vi "Update Inverter Data in MeasDataQ.vi"(6 "UpdateTS (T)":bool=TRUE, 8 "error in (no error)":errorcluster, 9 "TimeStamp":timestamp, 11 "Inverter Data":T1) -> (0 "error out":errorcluster, 3 "InverterWaveformsQ out":T2)   [LabVIEW 2019]
doc: "Developed by Kevin Thompson\nThompson Engineering, LLC\nkevin@thompsonengineering.net"
uses:
  TD MeasData--cluster.ctl
  TD MeasData QRef.ctl
  GBL DataQ Ref.vi
  DataTypes/InverterData--cluster.ctl
  DataTypes/InverterPhaseData--cluster.ctl
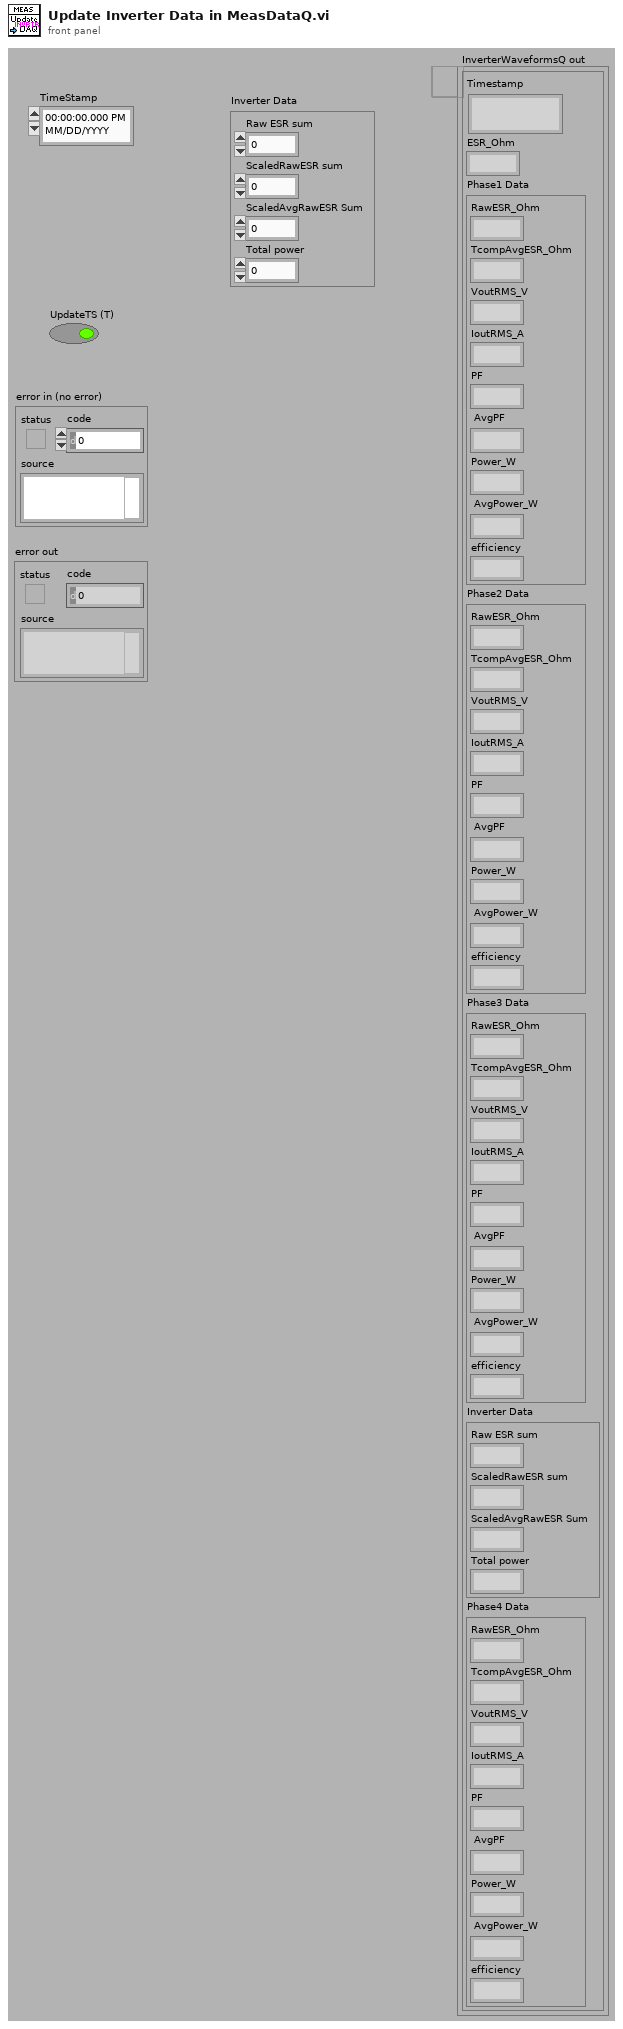
[diagram p1: front panel]
types:
  T1 = typedef "InverterData--cluster.ctl" = cluster{"Raw ESR sum":dbl, "ScaledRawESR sum":dbl, "ScaledAvgRawESR Sum":dbl, "Total power":dbl}
  T2 = typedef "TD MeasData QRef.ctl" = refnum<queue>
  T3 = typedef "TD MeasData--cluster.ctl" = cluster{"Timestamp":timestamp, "ESR_Ohm":dbl, "Phase1 Data":T4, "Phase2 Data":T4, "Phase3 Data":T4, "Inverter Data":T1, "Phase4 Data":T4}
  T4 = typedef "InverterPhaseData--cluster.ctl" = cluster{"RawESR_Ohm":dbl, "TcompAvgESR_Ohm":dbl, "VoutRMS_V":dbl, "IoutRMS_A":dbl, "PF":dbl, "AvgPF":dbl, "Power_W":dbl, "AvgPower_W":dbl, "efficiency":dbl}
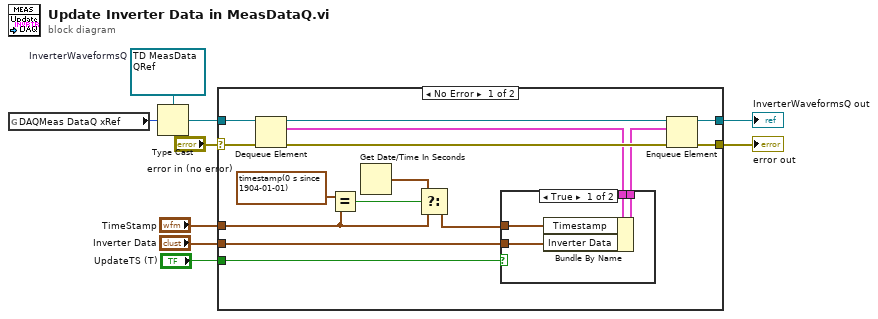
[diagram p0: block diagram]
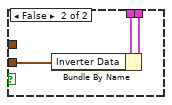
[diagram p2: hidden frame]
diagram:
  w6 = T2 refnum  # InverterWaveformsQ
  n1 = global read "GBL DataQ Ref.vi" "DAQMeas DataQ xRef"() -> (w3:u32)
  n2 = Type Cast(type=w6, x=w3) -> (*(type *) &x=w5:T2)
  n3 = case shown="No Error" "error in (no error)" {
    selector: "error in (no error)" -> [w19 w32]
    tunnel: w5 -> [w24 w33]
    tunnel: [w21 w32] -> w9
    tunnel: [w20 w33] -> w8
    tunnel: "TimeStamp" -> [w14 _]
    tunnel: "Inverter Data" -> [w10 _]
    tunnel: "UpdateTS (T)" -> [w11 _]
    frame No Error {
      n4 = Dequeue Element(queue=w24, error in (no error)=w19) -> (queue out=w22:T2, element=w18:T3, error out=w23:errorcluster)  [unwired: 1 in, 1 out]
      n5 = Equal?(x=timestamp(0 s since 1904-01-01) ("TimeStamp"), y=w14) -> (x = y?=w15:bool)
      n6 = Get Date/Time In Seconds() -> (seconds since 1Jan1904=w12:timestamp)
      n7 = Select(t=w12, s=w15, f=w14) -> (s? t:f=w13:timestamp)
      n8 = case shown="True" w11 {
        tunnel: w18 -> [w28 w31]
        tunnel: [w27 w30] -> w17
        tunnel: w13 -> [w26 _]
        tunnel: w10 -> [w25 w29]
        frame True {
          n9 = Bundle By Name(cluster=w28, "Timestamp"=w26, "Inverter Data"=w25) -> (w27:T3)
        }
        frame False {
          n10 = Bundle By Name(cluster=w31, "Inverter Data"=w29) -> (w30:T3)
        }
      }
      n11 = Enqueue Element(queue=w22, element=w17, error in (no error)=w23) -> (queue out=w20:T2, error out=w21:errorcluster)  [unwired: 1 in, 1 out]
    }
    frame Error {
    }
  }
  "InverterWaveformsQ out" <- w8
  "error out" <- w9
